vi "TREE_Test.vi"(7 "Label":string="Tree", 8 "error in":errorcluster, 11 "VI Server.RefsCluster":T3) -> (0 "error out":errorcluster={"status"=TRUE, "code"=1077, "source"="Property Node (arg 1) in VI Server_TREE_ItemSymbol_SET.vi->TREE_Test.vi\n<APPEND>\nProperty Name: <b>Active Item:Row Number</b>"}, 3 "VI Server.RefsCluster.DUP":T3)   [LabVIEW 2020]
uses:
  VI Server_TypeDefs/VI Server_RefsCluster.ctl
  VI Server_TypeDefs/VI Server_Tree_Items.ctl
  VI Server_TypeDefs/VI Server_TREE_ActiveCell_Pos.ctl
panel:
  in  "Text":string
  in  "AciveCell.Position":T1={"Row Number\n(-2-all clmns)"=0, "Column Number\n(-2 - whole row)"=3} {"Column Number\n(-2 - whole row)" min=-2}
  in  "Active Cell:Active Column Number 2":i32=3
  in  "BG.Color":u32(colorbox)
  in  "Column Header Strings[]":T2[](array[typedef])=[{"LeftCell.String"="First Cell", "Child.Text"=[], "Child.Tag"="", "ItemIndent.Level"=0}, {"LeftCell.String"="First Cild", "Child.Text"=[], "Child.Tag"="", "ItemIndent.Level"=1}, {"LeftCell.String"="Second Child", "Child.Text"=["2ndChils"], "Child.Tag"="", "ItemIndent.Level"=1}, {"LeftCell.String"="3rdCild", "Child.Text"=["3rdChild_Txt"], "Child.Tag"="", "ItemIndent.Level"=2}]
  in  "Tree":string(tree)="Duplicate Tag_1"
  in  "Stop Button":bool
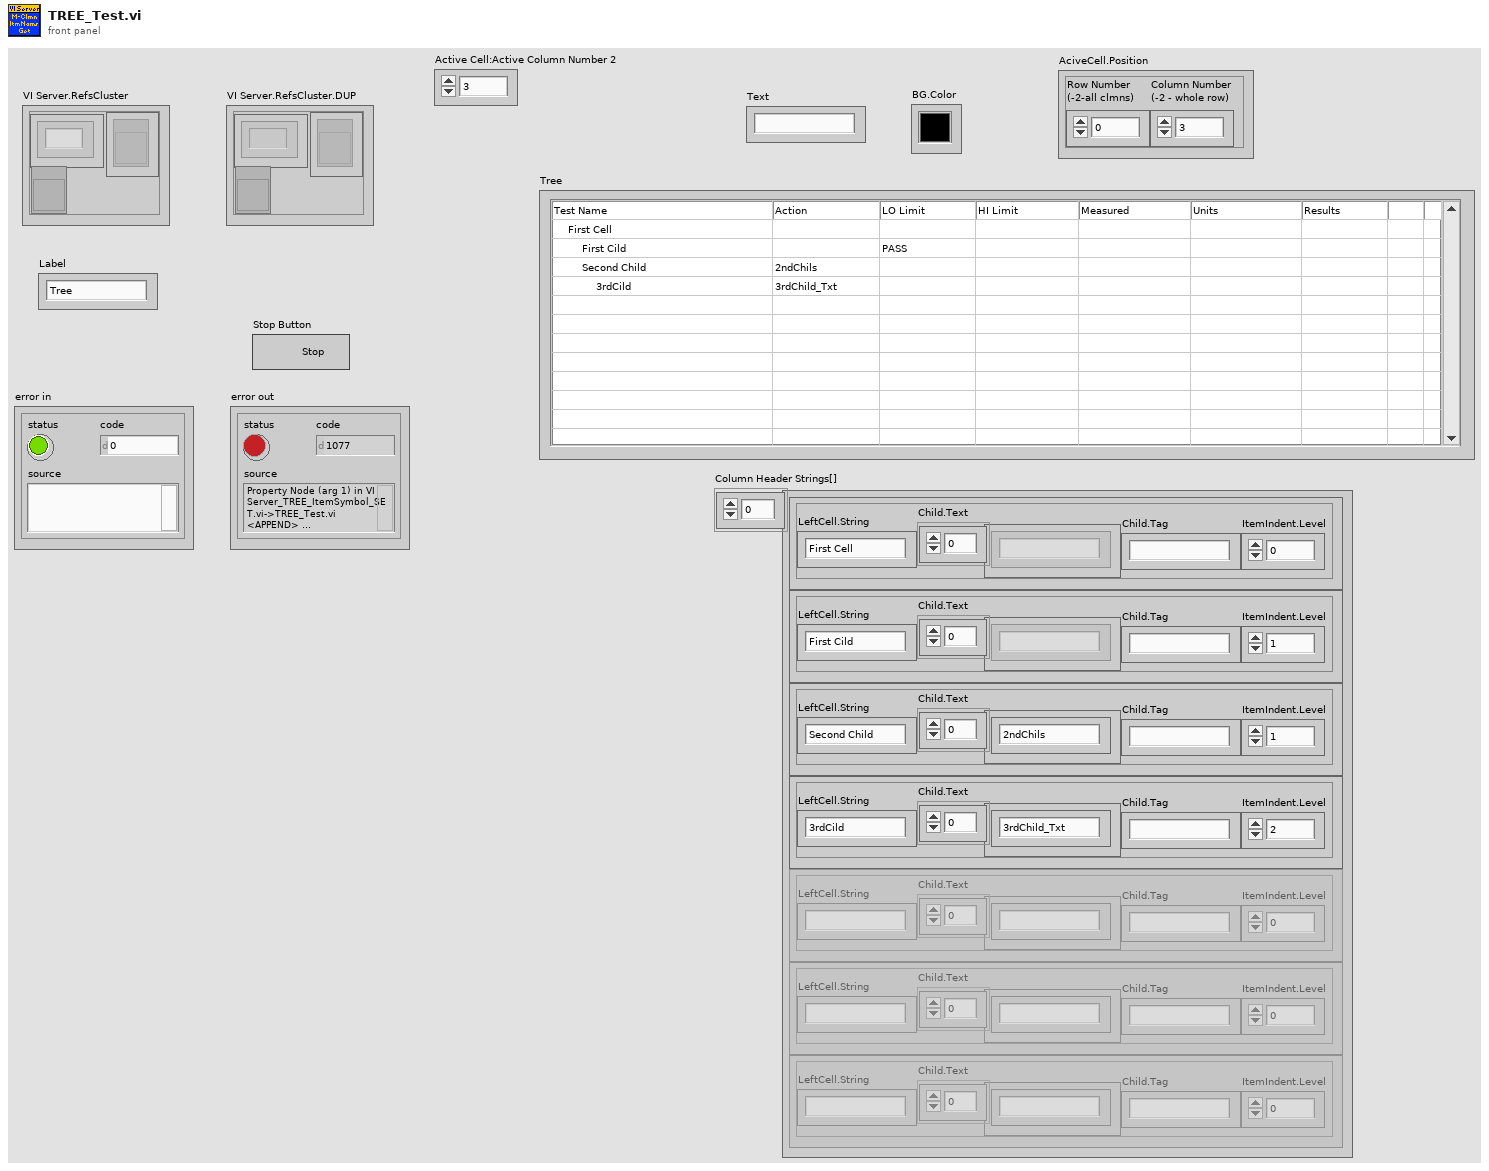
[diagram p1: front panel]
types:
  T1 = typedef "VI Server_TREE_ActiveCell_Pos.ctl" = cluster{"Row Number\n(-2-all clmns)":i32, "Column Number\n(-2 - whole row)":i32}
  T2 = typedef "VI Server_Tree_Items.ctl" = cluster{"LeftCell.String":string, "Child.Text":string[], "Child.Tag":string, "ItemIndent.Level":i32}
  T3 = typedef "VI Server_RefsCluster.ctl" = cluster{"Labels":string[], "Refs":refnum<vi>[], "VI Ref":refnum<vi>}
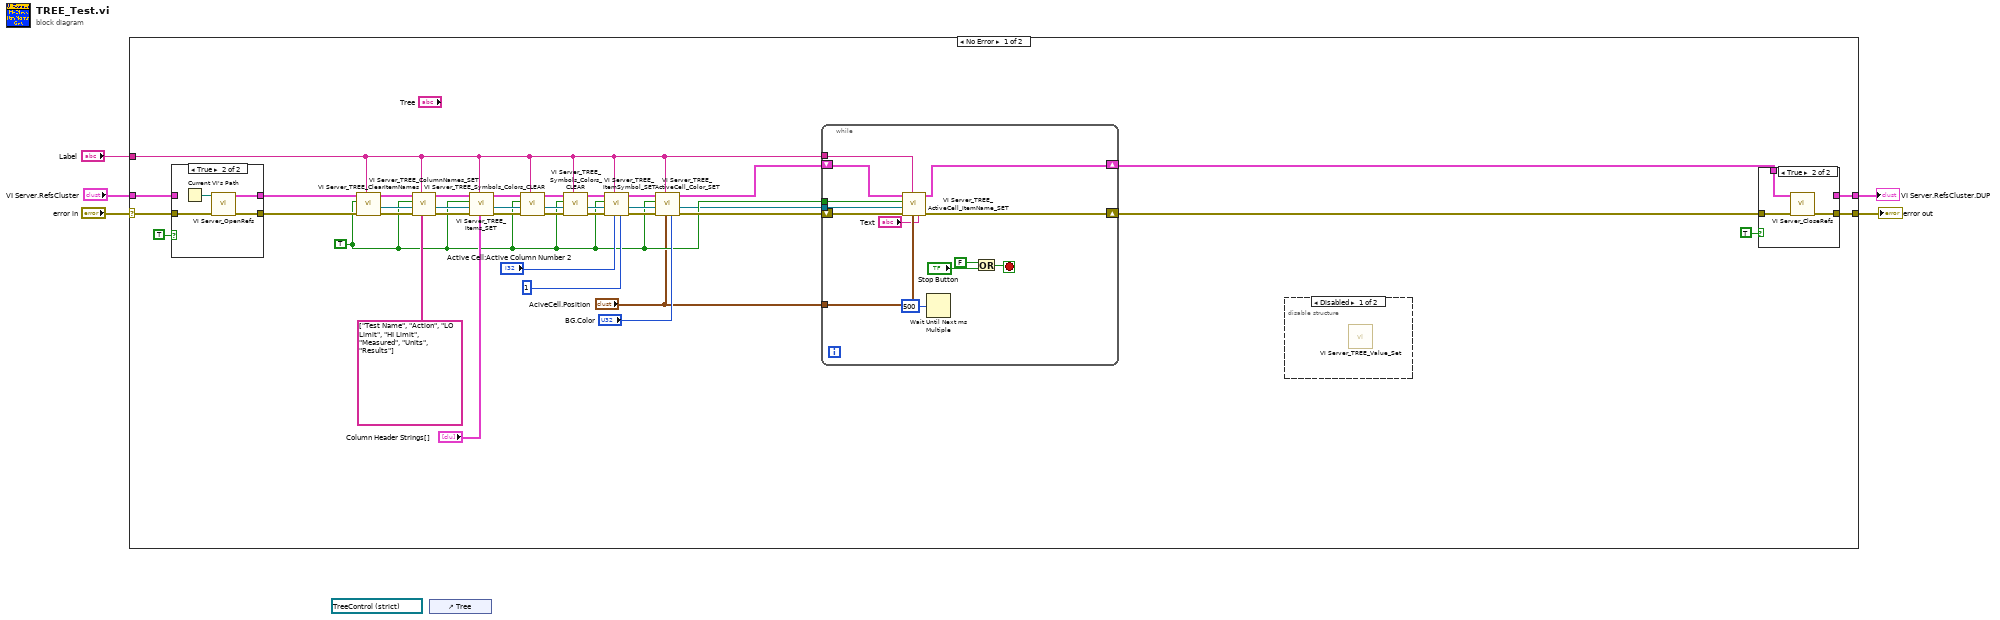
[diagram p0: block diagram]
diagram:
  (unwired) refnum<vi> refnum ("Tree")
  n1 = case shown="No Error" "error in" {
    selector: "error in" -> [w44 w70]
    tunnel: [w41 w70] -> w4
    tunnel: "VI Server.RefsCluster" -> [w42 w69]
    tunnel: [w39 w69] -> w2
    tunnel: "Label" -> [w9 _]
    frame No Error {
      w8 = TRUE ("SingleInstance")
      n2 = case shown="True" TRUE {
        tunnel: w44 -> [w64 w68]
        tunnel: [w64 w66] -> w38
        tunnel: [w63 w65] -> w17
        tunnel: w42 -> [w63 _]
        frame False {
        }
        frame True {
          n3 = Current VI's Path() -> (path=w67:path)
          n4 = call "VI Server_OpenRefs.vi"("error in"=w68, "VI Path"=w67) -> ("error out"=w66:errorcluster, "VI Server.RefsCluster"=w65:T3)  [unwired: 8 in]
        }
      }
      n5 = call "VI Server_TREE_ClearItemNames.vi"("Label"=w9, "error in"=w38, "SingleInstance"=w8, "VI Server.RefsCluster"=w17) -> ("error out"=w33:errorcluster, "Tree.Ref.DUP"=w31:refnum<vi>, "VI Server.RefsCluster.DUP"=w32:T3)  [unwired: 5 in]
      n6 = call "VI Server_TREE_ColumnNames_SET.vi"("Column Header Strings[]"=string[] ["Test Name", "Action", "LO Limit", "HI Limit", "Measured", "Units", "Results"], "Label"=w9, "error in"=w33, "Tree.Ref"=w31, "SingleInstance"=w8, "VI Server.RefsCluster"=w32) -> ("error out"=w36:errorcluster, "Tree.Ref.DUP"=w30:refnum<vi>, "VI Server.RefsCluster.DUP"=w35:T3)  [unwired: 3 in]
      n7 = call "VI Server_TREE_Items_SET.vi"("Column Header Strings[]"="Column Header Strings[]", "Label"=w9, "error in"=w36, "Tree.Ref"=w30, "SingleInstance"=w8, "VI Server.RefsCluster"=w35) -> ("error out"=w29:errorcluster, "Tree.Ref"=w27:refnum<vi>, "VI Server.RefsCluster.DUP"=w28:T3)  [unwired: 3 in]
      n8 = call "VI Server_TREE_Symbols_Colors_CLEAR.vi"("Label"=w9, "error in"=w29, "Tree.Ref"=w27, 10:w8, "VI Server.RefsCluster"=w28) -> ("error out"=w26:errorcluster, "Tree.Ref.DUP"=w24:refnum<vi>, "VI Server.RefsCluster.DUP"=w25:T3)  [unwired: 4 in]
      n9 = call "VI Server_TREE_Symbols_Colors_CLEAR.vi"("Label"=w9, "error in"=w26, "Tree.Ref"=w24, 10:w8, "VI Server.RefsCluster"=w25) -> ("error out"=w23:errorcluster, "Tree.Ref.DUP"=w22:refnum<vi>, "VI Server.RefsCluster.DUP"=w21:T3)  [unwired: 4 in]
      n10 = call "VI Server_TREE_ItemSymbol_SET.vi"("Symbol"=1, "Active Cell:Active Column Number"="Active Cell:Active Column Number 2", "Label"=w9, "error in"=w23, "Tree.Ref"=w22, "SingleInstance"=w8, "VI Server.RefsCluster"=w21) -> ("error out"=w18:errorcluster, "Tree.Ref.DUP"=w16:refnum<vi>, "VI Server.RefsCluster.DUP"=w15:T3)  [unwired: 2 in]
      n11 = call "VI Server_TREE_ActiveCell_Color_SET.vi"("BG.Color"="BG.Color", "AciveCell.Position"="AciveCell.Position", "Label"=w9, "error in"=w18, "Tree.Ref"=w16, "SingleInstance"=w8, "VI Server.RefsCluster"=w15) -> ("error out"=w13:errorcluster, "Tree.Ref.DUP"=w7:refnum<vi>, "VI Server.RefsCluster.DUP"=w11:T3)  [unwired: 2 in]
      n12 = while {
        tunnel: w9 -> [w50]
        tunnel: w8 -> [w49]
        tunnel: w7 -> [w48]
        tunnel: "AciveCell.Position" -> [w47]
        shift-right: [w53] -> w12
        shift-left: w13 -> [w54]
        shift-right: [w51] -> w10
        shift-left: w11 -> [w52]
        stop <- w46 stop-if-true
        n13 = call "VI Server_TREE_ActiveCell_ItemName_SET.vi"("Text"="Text", "AciveCell.Position"=w47, "Label"=w50, "error in"=w54, "Tree.Ref"=w48, "SingleInstance"=w49, "VI Server.RefsCluster"=w52) -> ("error out"=w53:errorcluster, "VI Server.RefsCluster.DUP"=w51:T3)  [unwired: 2 in, 1 out]
        n14 = Wait Until Next ms Multiple(millisecond multiple=u32 500) -> ()  [unwired: 1 out]
        n15 = Or(x=FALSE, y="Stop Button") -> (x .or. y?=w46:bool)
      }
      n16 = disable-structure shown="Disabled" {
        frame Disabled {
          n17 = call "VI Server_TREE_Value_Set.vi"() -> ()  [unwired: 9 in, 3 out]
        }
        frame Enabled {
        }
      }
      n18 = case shown="True" TRUE {
        tunnel: w12 -> [w59 w62]
        tunnel: [w59 w61] -> w41
        tunnel: w10 -> [w58 w60]
        tunnel: [w58 _] -> w39
        frame False {
        }
        frame True {
          n19 = call "VI Server_CloseRefs.vi"("error in"=w62, "VI Server.RefsCluster"=w60) -> ("error out"=w61:errorcluster)  [unwired: 9 in]
        }
      }
    }
    frame Error {
    }
  }
  "VI Server.RefsCluster.DUP" <- w2
  "error out" <- w4
  n20 = control-ref of="Tree"() -> ()  [unwired: 1 out]
